vi "SSIToolMain.vi"() -> ()   [LabVIEW 2019]
uses:
  testSeq/TestSeqClass.lvclass
  Exe_Queues/TypeDef/mainExeStates.ctl
  Exe_Queues/TypeDef/mainEventInfo.ctl
  GUIHandler/GUI_Handler_Seq.lvclass
  GUIHandler_Main/GUI_Handler_Main.lvclass
  GUIHandler/GuiSectionEnum.ctl
  Typedef/TestTypeSelect.ctl
  ProgramSettings/ProgramSettings.lvclass
panel:
  in  "Calibration_ListBox":i32(listbox)=-1
  in  "Operatør beskeder":T1={"Operator_Aceept"=FALSE, "Operator_decline "=FALSE, "User message "="Er Lysdioden slukket"}
  in  "Forsyningsspænding":u16(ring)=1 items=["", "5V", "9 - 30 V"]
  out "Calibration Status":bool=TRUE
  out "Multiturn værdi":dbl
  out "Singleturn værdi":dbl
  out "Test Status":bool=TRUE
  in  "Test_Listbox":i32(listbox)=-1
  in  "Kode":u16(ring)=2 items=["", "Binær", "Gray"]
  in  "Opløsning":u16(ring)=2 items=["", "0013", "1213", "1613", "2013", "2413"]
  in  "Konfigurations Filnavn":string="Test.cfg"
  out "Dial":dbl(knob)=0.604351805313778 scale=0.0..360.0
  in  "StartCalibration":bool
  in  "StartAfprøvning":bool
  in  "Start Alt":bool
  in  "Stop":bool
  # "Variant setup"
  # "Konfiguration"
  # "Afprøvning"
  # "Aktuelle værdier"
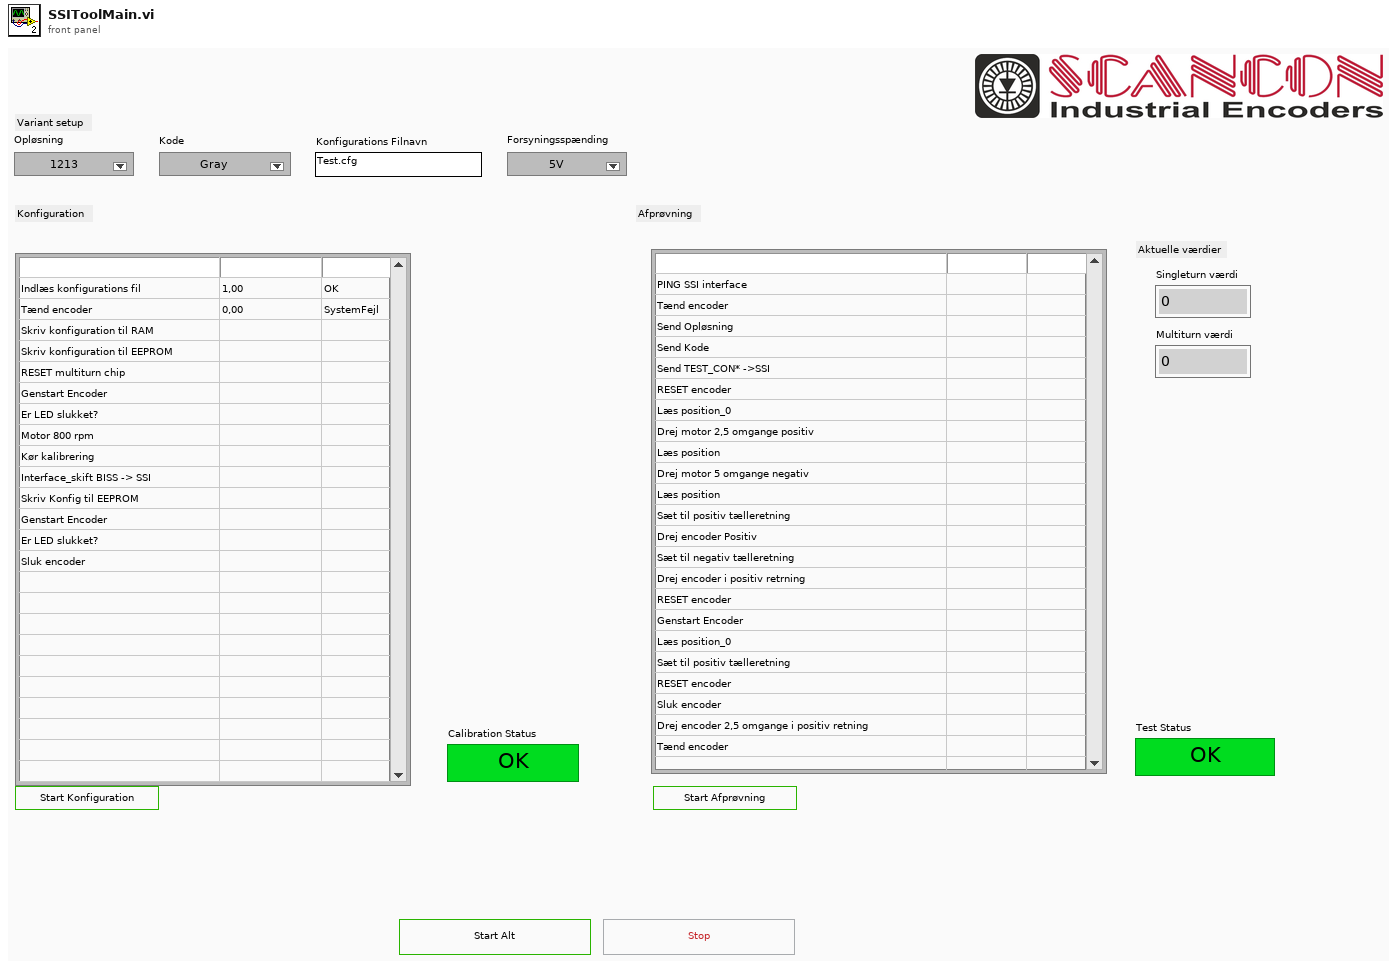
[diagram p1: front panel]
types:
  T1 = cluster{"Operator_Aceept":bool, "Operator_decline ":bool, "User message ":string}
  T2 = cluster{"Start Alt":refnum<vi>, "Stop":refnum<vi>, "Operatør beskeder":refnum<vi>}
  T3 = typedef "GuiSectionEnum.ctl" = enum16{"TestingSection", "CalibrationSection"}
  T4 = cluster{"Konfigurations Filnavn":refnum<vi>, "Forsyningsspænding":refnum<vi>, "Kode":refnum<vi>, "Opløsning":refnum<vi>}
  T5 = typedef "mainEventInfo.ctl" = cluster{"MainExeStates":T6, "Data":variant}
  T6 = typedef "mainExeStates.ctl" = enum16{"Idle", "Load_Seq_File", "Save_Seq_File", "Init", "StartKalib", "StartAfprøvning", "StartAlt", "Stop", "Exit", "SettingsDialog", "Update_Config_FileName", "Seq_Calibrate_setup"}
  T7 = cluster{"Multiturn værdi":refnum<vi>, "Singleturn værdi":refnum<vi>, "Test Status":refnum<vi>, "Test_Listbox":refnum<vi>, "Dial":refnum<vi>, "StartAfprøvning":refnum<vi>}
  T8 = typedef "TestTypeSelect.ctl" = enum16{"Calibration", "Testing"}
  T9 = cluster{"MHM_Handle out":u32, "axis out":cluster{"keyHandle":u32, "nodeId":u16}}
  T10 = enum32{"invalid app kind", "Development System", "Run Time System", "Student Edition", "Embedded LabVIEW", "Evaluation", "Custom"}
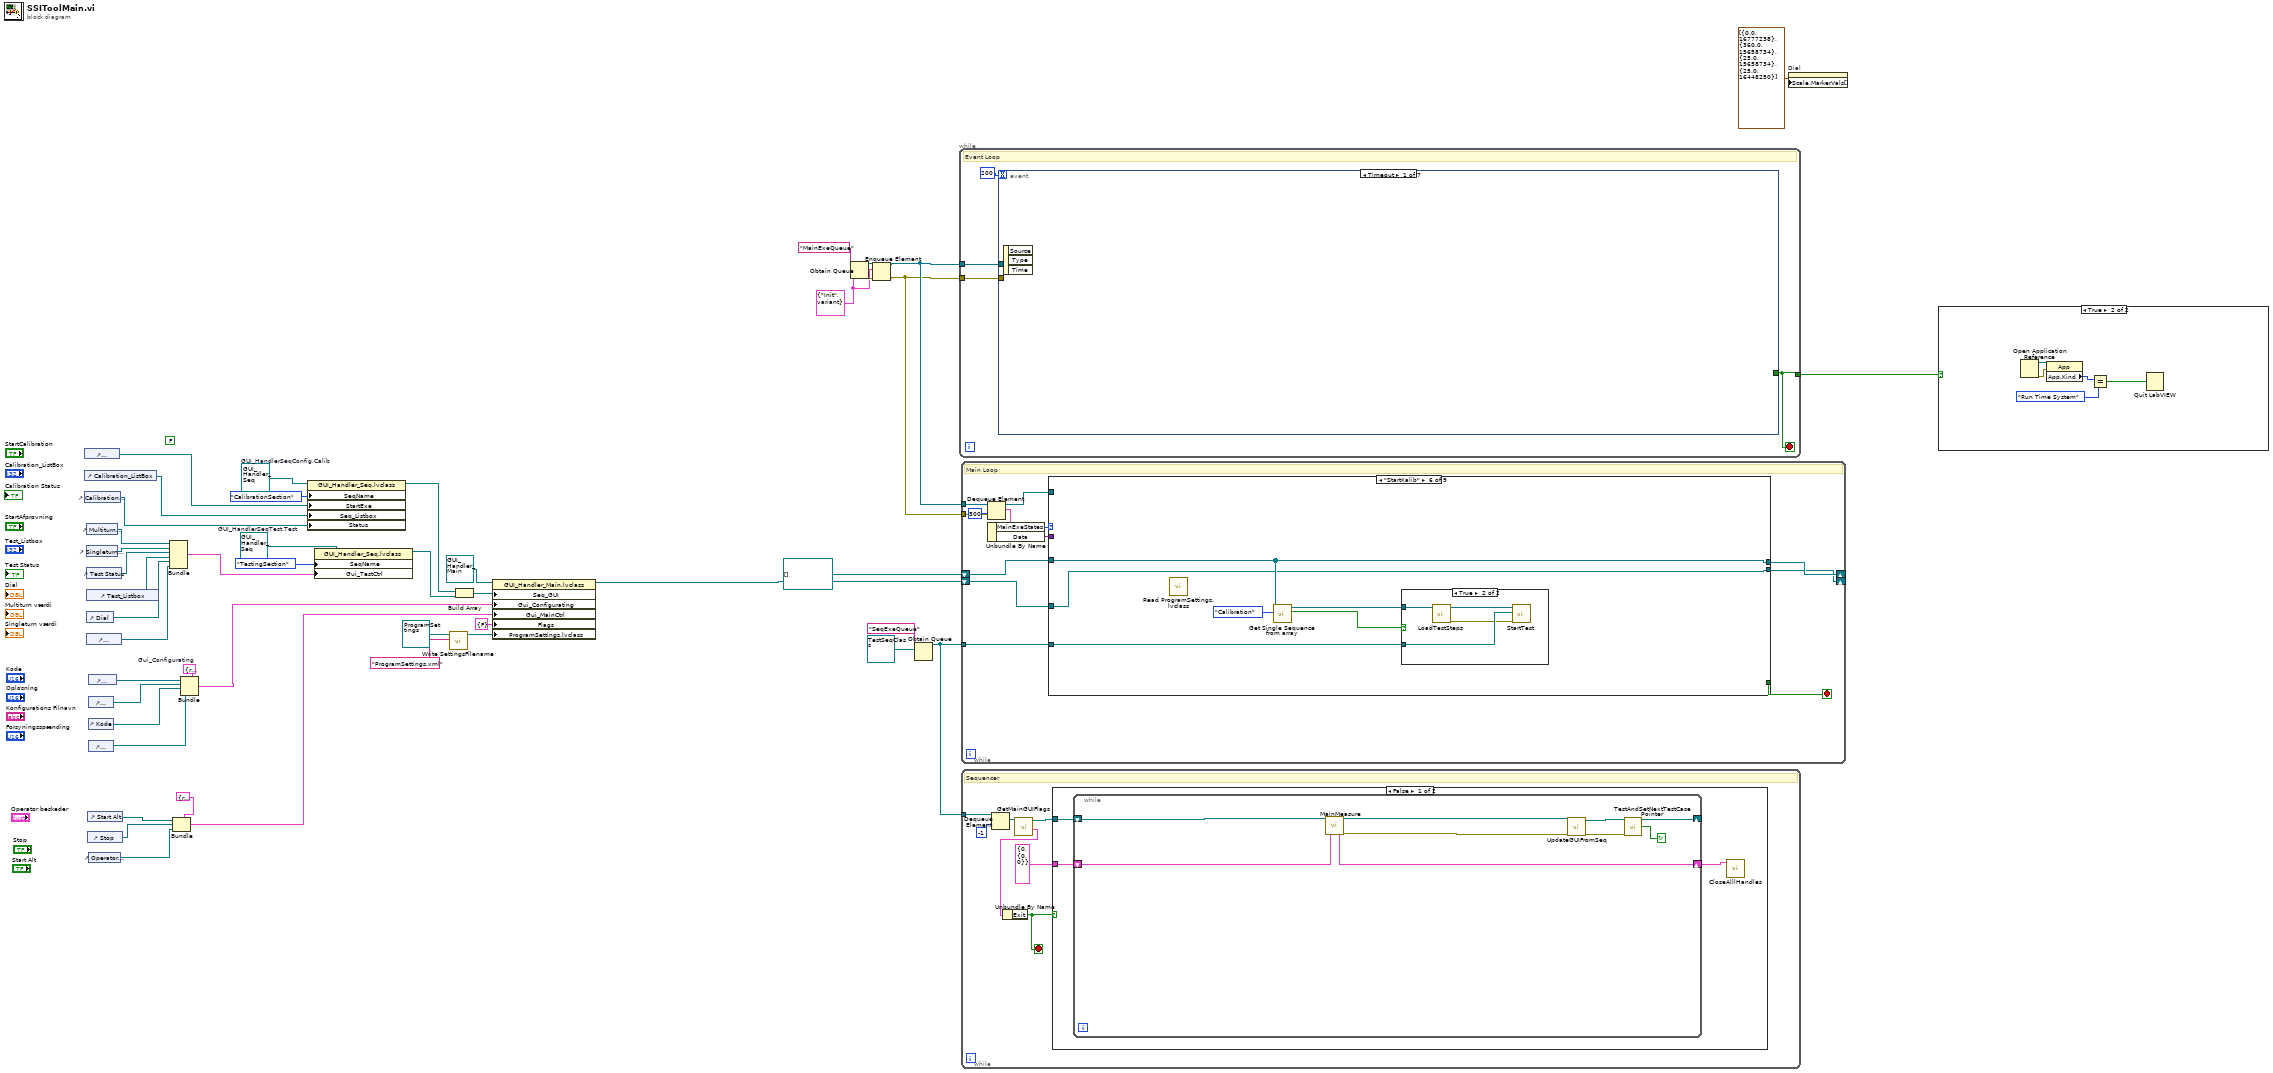
[diagram p0: block diagram]
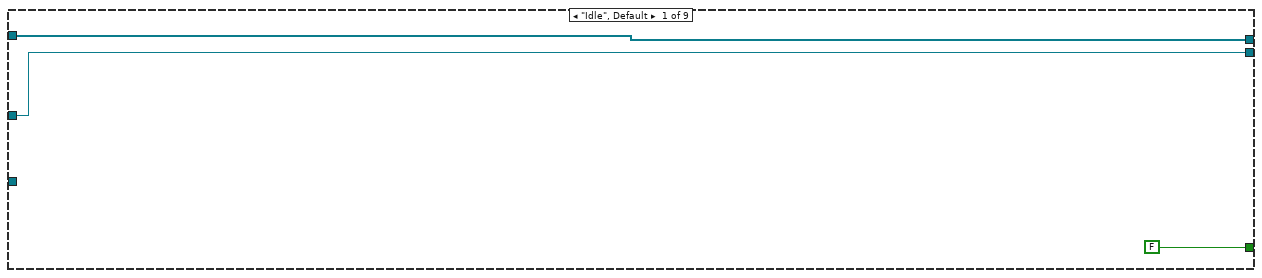
[diagram p4: hidden frame]
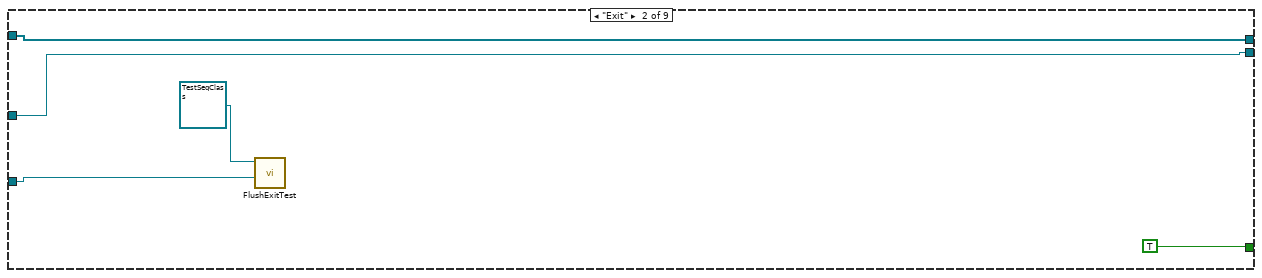
[diagram p5: hidden frame]
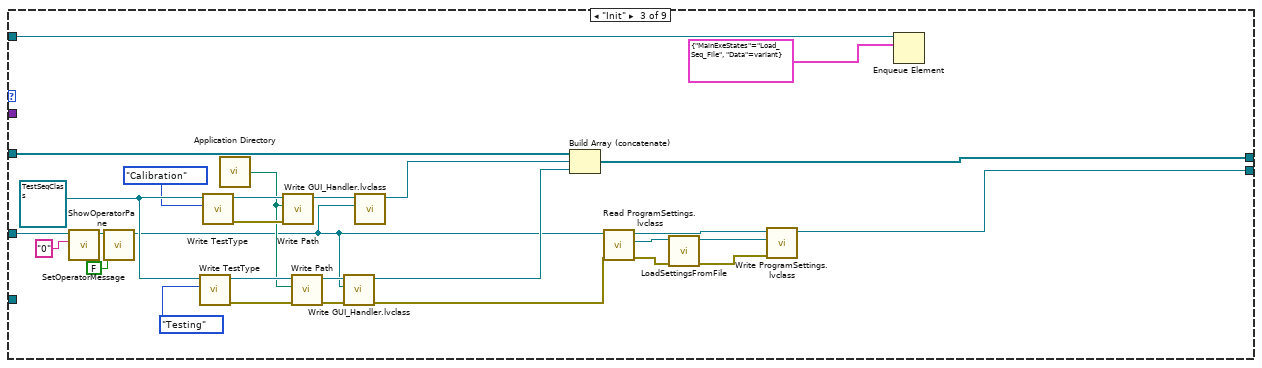
[diagram p6: hidden frame]
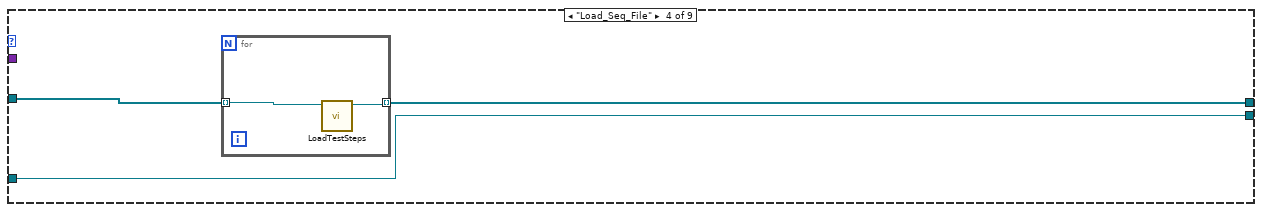
[diagram p7: hidden frame]
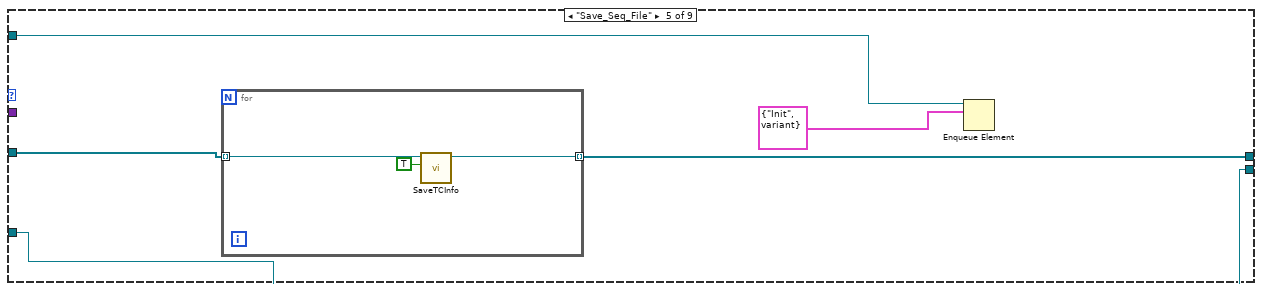
[diagram p8: hidden frame]
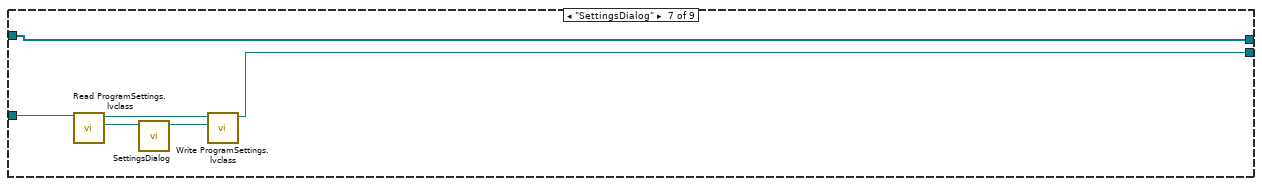
[diagram p10: hidden frame]
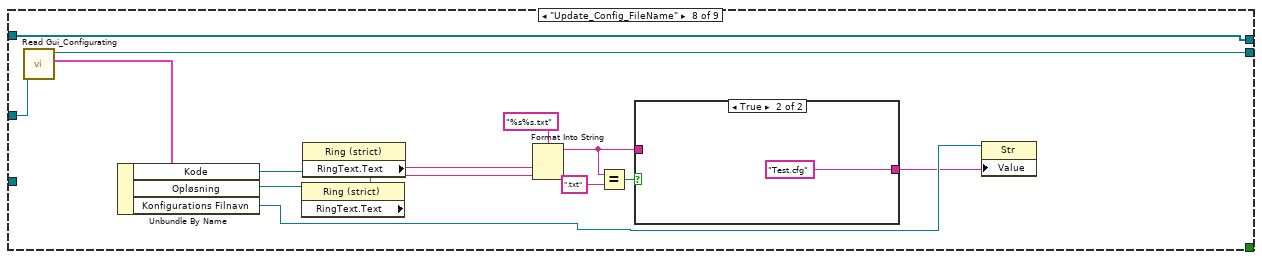
[diagram p11: hidden frame]
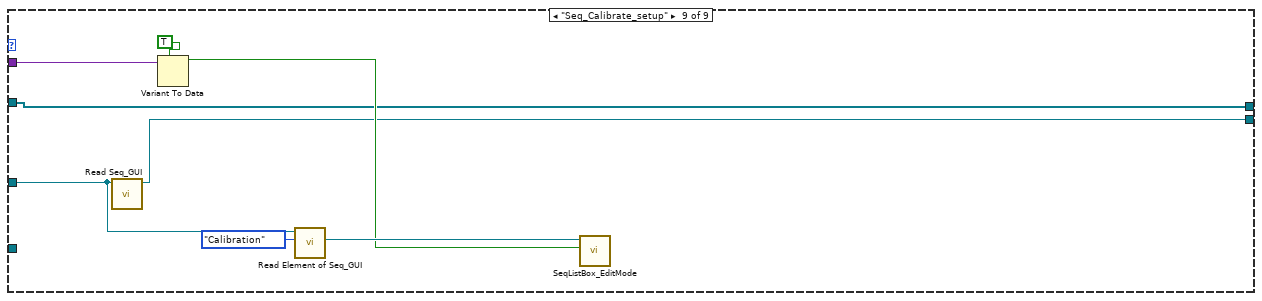
[diagram p13: hidden frame]
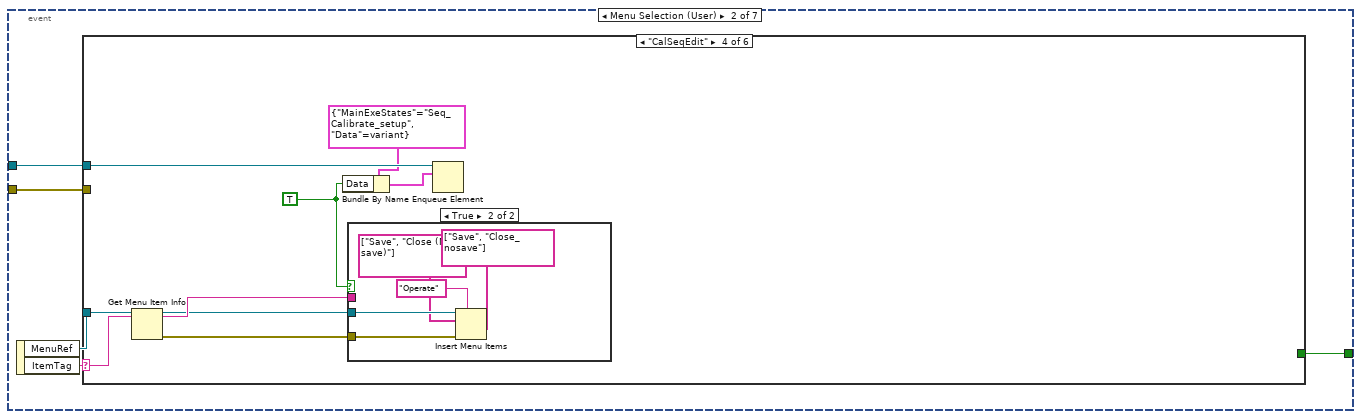
[diagram p14: hidden frame]
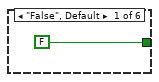
[diagram p15: hidden frame]
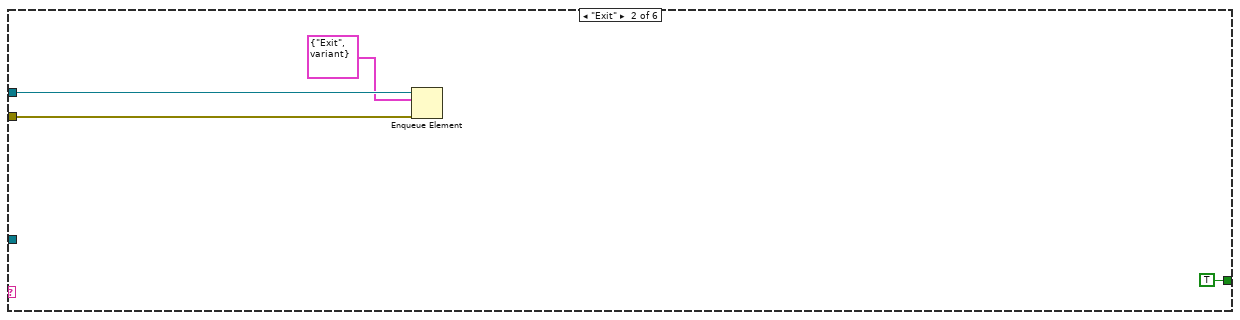
[diagram p16: hidden frame]
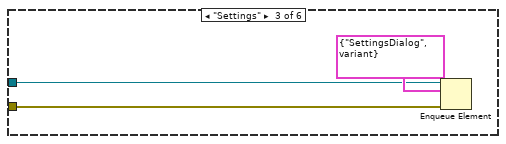
[diagram p17: hidden frame]
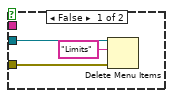
[diagram p18: hidden frame]
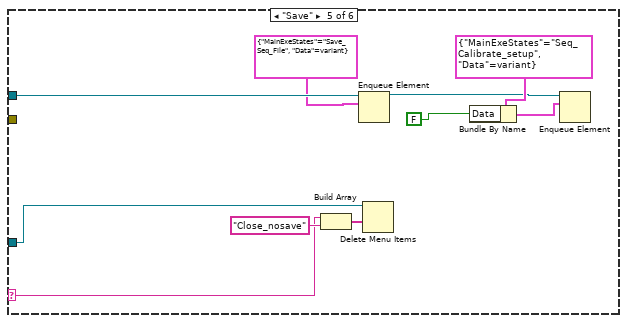
[diagram p19: hidden frame]
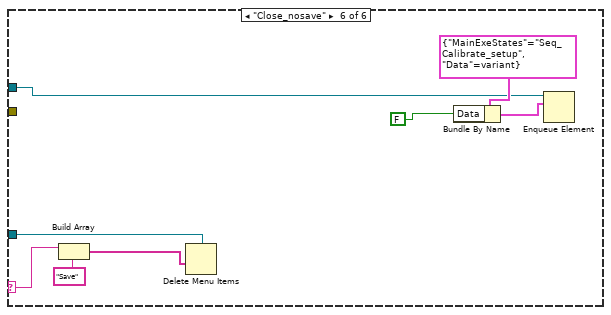
[diagram p20: hidden frame]
diagram:
  (unwired) FALSE ("Blinking")
  w26 = T4 {"Konfigurations Filnavn"=refnum, "Forsyningsspænding"=refnum, "Kode"=refnum, "Opløsning"=refnum}  # Gui_Configurating
  w20 = refnum<class "GUI_Handler_Seq.lvclass"> refnum  # GUI_HandlerSeqTest.Test
  w39 = T5 {"MainExeStates"=enum."Init", "Data"=variant}
  w25 = refnum<class "GUI_Handler_Seq.lvclass"> refnum  # GUI_HandlerSeqConfig.Calib
  n1 = control-ref of="StartCalibration"() -> (w23:refnum<vi>)
  n2 = control-ref of="Calibration_ListBox"() -> (w22:refnum<vi>)
  n3 = control-ref of="Calibration Status"() -> (w10:refnum<vi>)
  n4 = control-ref of="Multiturn værdi"() -> (w32:refnum<vi>)
  n5 = control-ref of="Singleturn værdi"() -> (w31:refnum<vi>)
  n6 = control-ref of="Test Status"() -> (w30:refnum<vi>)
  n7 = control-ref of="Test_Listbox"() -> (w29:refnum<vi>)
  n8 = control-ref of="Dial"() -> (w28:refnum<vi>)
  n9 = control-ref of="StartAfprøvning"() -> (w27:refnum<vi>)
  n10 = control-ref of="Stop"() -> (w3:refnum<vi>)
  n11 = control-ref of="Start Alt"() -> (w4:refnum<vi>)
  n12 = control-ref of="Konfigurations Filnavn"() -> (w36:refnum<vi>)
  n13 = control-ref of="Forsyningsspænding"() -> (w35:refnum<vi>)
  n14 = control-ref of="Kode"() -> (w34:refnum<vi>)
  n15 = control-ref of="Opløsning"() -> (w33:refnum<vi>)
  n16 = control-ref of="Operatør beskeder"() -> (w2:refnum<vi>)
  n17 = Bundle("Multiturn værdi"=w32, "Singleturn værdi"=w31, "Test Status"=w30, "Test_Listbox"=w29, "Dial"=w28, "StartAfprøvning"=w27) -> (w19:T7)  [unwired: 1 in]
  n18 = Bundle(cluster=T2 {"Start Alt"=refnum, "Stop"=refnum, "Operatør beskeder"=refnum} ("output cluster"), "Start Alt"=w4, "Stop"=w3, "Operatør beskeder"=w2) -> (w5:T2)
  n19 = Bundle(cluster=w26, "Konfigurations Filnavn"=w36, "Forsyningsspænding"=w35, "Kode"=w34, "Opløsning"=w33) -> (w16:T4)
  n20 = property class="GUI_Handler_Seq.lvclass"(reference=w25, "SeqName"=GuiSectionEnum."CalibrationSection", "StartExe"=w23, "Seq_Listbox"=w22, "Status"=w10) -> (reference out=w43:refnum<class "GUI_Handler_Seq.lvclass">)  [unwired: 1 in, 1 out]
  n21 = property class="GUI_Handler_Seq.lvclass"(reference=w20, "SeqName"=GuiSectionEnum."TestingSection", "Gui_TestCtrl"=w19) -> (reference out=w42:refnum<class "GUI_Handler_Seq.lvclass">)  [unwired: 1 in, 1 out]
  n22 = call "Write SettingsFilename.vi"("SettingsFilename"="ProgramSettings.xml", "ProgramSettings in"=refnum<class "ProgramSettings.lvclass"> refnum ("ProgramSettings.lvclass")) -> ("ProgramSettings out"=w7:refnum<class "ProgramSettings.lvclass">)  [unwired: 8 in, 1 out]
  n23 = Build Array(w43, w42) -> (w17:refnum<class "GUI_Handler_Seq.lvclass">[])
  n24 = property class="GUI_Handler_Main.lvclass"(reference=refnum<class "GUI_Handler_Main.lvclass"> refnum ("GUI_Handler_Main.lvclass"), "Seq_GUI"=w17, "Gui_Configurating"=w16, "Gui_MainCtrl"=w5, "Flags"=cluster{"Exit":bool} {"Exit"=FALSE}, "ProgramSettings.lvclass"=w7) -> (reference out=w15:refnum<class "GUI_Handler_Main.lvclass">)  [unwired: 1 in, 1 out]
  n25 = Obtain Queue(name (unnamed)="MainExeQueue", element data type=w39) -> (queue out=w41:refnum<queue>, error out=w40:errorcluster)  [unwired: 3 in, 1 out]
  n26 = Enqueue Element(queue=w41, element=w39, error in (no error)=w40) -> (queue out=w38:refnum<queue>, error out=w37:errorcluster)  [unwired: 1 in, 1 out]
  n27 = Obtain Queue(name (unnamed)="SeqExeQueue", element data type=refnum<class "TestSeqClass.lvclass"> refnum ("TestSeqClass.lvclass")) -> (queue out=w11:refnum<queue>)  [unwired: 3 in, 2 out]
  n28 = while {
    tunnel: [w49] -> w45
    tunnel: w38 -> [w48]
    tunnel: w37 -> [w47]
    stop <- w49 stop-if-true
    # "Event Loop"
    n29 = event shown="[0] Timeout" {
      selector: _ -> [_ _ _ _ _ _ _]
      dyn-events: _ -> [_ _ _ _ _ _ _]
      timeout: 200 -> [_ _ _ _ _ _ _]
      tunnel: [_ w54 _ _ _ _ _] -> w49
      tunnel: w48 -> [_ w53 w99 w101 w104 w110 _]
      tunnel: w47 -> [_ w52 w98 _ w103 w109 _]
      event Timeout {
        n30 = event-data() -> ()  [unwired: 1 in, 3 out]
      }
      event Menu Selection (User) {
        n31 = event-data() -> ("MenuRef"=w51:refnum<k9>, "ItemTag"=w55:string)  [unwired: 1 in]
        n32 = case shown="\"CalSeqEdit\"" w55 {
          selector: w55 -> [_ _ _ w67 w85 w92]
          tunnel: [FALSE TRUE _ _ _ _] -> w54
          tunnel: w53 -> [_ w59 w62 w71 w89 w96]
          tunnel: w52 -> [_ w58 w61 _ _ _]
          tunnel: w51 -> [_ _ _ w70 w84 w93]
          frame "False", Default {
          }
          frame "Exit" {
            n33 = Enqueue Element(queue=w59, element=T5 {"MainExeStates"=enum."Exit", "Data"=variant}, error in (no error)=w58) -> ()  [unwired: 1 in, 3 out]
          }
          frame "Settings" {
            n34 = Enqueue Element(queue=w62, element=T5 {"MainExeStates"=enum."SettingsDialog", "Data"=variant}, error in (no error)=w61) -> ()  [unwired: 1 in, 3 out]
          }
          frame "CalSeqEdit" {
            w64 = TRUE
            n35 = Get Menu Item Info(7:w67, 11:w70) -> (0:w65:errorcluster, 3:w66:refnum<k9>)  [unwired: 1 in, 5 out]
            n36 = Bundle By Name(cluster=T5 {"MainExeStates"=enum."Seq_Calibrate_setup", "Data"=variant} ("element"), "Data"=w64) -> (w68:T5)
            n37 = case shown="True" w64 {
              tunnel: w65 -> [w74 w79]
              tunnel: w66 -> [w73 w78]
              tunnel: w67 -> [_ _]
              frame False {
                n38 = Delete Menu Items(6:w74, 8:"Limits" ("menu tag"), 9:w73) -> ()  [unwired: 1 in, 2 out]
              }
              frame True {
                n39 = Insert Menu Items(5:"Operate" ("menu tag"), 6:w79, 7:string[] ["Save", "Close_nosave"] ("item tags"), 8:string[] ["Save", "Close (No save)"] ("item names"), 9:w78) -> ()  [unwired: 1 in, 3 out]
              }
            }
            n40 = Enqueue Element(queue=w71, element=w68) -> ()  [unwired: 2 in, 3 out]
          }
          frame "Save" {
            n41 = Build Array(w85, "Close_nosave" ("element")) -> (w87:string[])
            n42 = Enqueue Element(queue=w89, element=T5 {"MainExeStates"=enum."Save_Seq_File", "Data"=variant}) -> (queue out=w80:refnum<queue>)  [unwired: 2 in, 2 out]
            n43 = Delete Menu Items(7:w87, 9:w84) -> ()  [unwired: 2 in, 2 out]
            n44 = Bundle By Name(cluster=T5 {"MainExeStates"=enum."Seq_Calibrate_setup", "Data"=variant} ("element"), "Data"=FALSE) -> (w81:T5)
            n45 = Enqueue Element(queue=w80, element=w81) -> ()  [unwired: 2 in, 3 out]
          }
          frame "Close_nosave" {
            n46 = Build Array(w92, "Save" ("element")) -> (w91:string[])
            n47 = Delete Menu Items(7:w91, 9:w93) -> ()  [unwired: 2 in, 2 out]
            n48 = Bundle By Name(cluster=T5 {"MainExeStates"=enum."Seq_Calibrate_setup", "Data"=variant} ("element"), "Data"=FALSE) -> (w94:T5)
            n49 = Enqueue Element(queue=w96, element=w94) -> ()  [unwired: 2 in, 3 out]
          }
        }
      }
      event "Opløsning", "Kode": Value Change {
        n50 = event-data() -> ()  [unwired: 1 in, 5 out]
        n51 = Enqueue Element(queue=w99, element=T5 {"MainExeStates"=enum."Update_Config_FileName", "Data"=variant}, error in (no error)=w98) -> ()  [unwired: 1 in, 3 out]
      }
      event "StartAfprøvning": Value Change {
        n52 = event-data() -> ()  [unwired: 1 in, 5 out]
        n53 = Enqueue Element(queue=w101, element=T5 {"MainExeStates"=enum."StartAfprøvning", "Data"=variant}) -> ()  [unwired: 2 in, 3 out]
      }
      event "StartCalibration": Value Change {
        n54 = event-data() -> ()  [unwired: 1 in, 5 out]
        n55 = Enqueue Element(queue=w104, element=T5 {"MainExeStates"=enum."StartKalib", "Data"=variant}, error in (no error)=w103) -> ()  [unwired: 1 in, 3 out]
      }
      event "Start Alt": Value Change {
        n56 = event-data() -> ()  [unwired: 1 in, 5 out]
        n57 = Enqueue Element(queue=w110, element=T5 {"MainExeStates"=enum."StartKalib", "Data"=variant}, error in (no error)=w109) -> (queue out=w107:refnum<queue>, error out=w106:errorcluster)  [unwired: 1 in, 1 out]
        n58 = Enqueue Element(queue=w107, element=T5 {"MainExeStates"=enum."StartAfprøvning", "Data"=variant}, error in (no error)=w106) -> ()  [unwired: 1 in, 3 out]
      }
      event "Operatør beskeder.Operator_Aceept": Value Change {
        n59 = event-data() -> ()  [unwired: 1 in, 5 out]
      }
    }
  }
  n60 = while {
    tunnel: w38 -> [w124]
    tunnel: w37 -> [w123]
    shift-right: [w119] -> _
    shift-left: refnum<class "TestSeqClass.lvclass">[] [] -> [w120]
    tunnel: w11 -> [w114]
    shift-right: [w113] -> _
    shift-left: w15 -> [w116]
    stop <- w115 stop-if-true
    # "Main Loop"
    n61 = Dequeue Element(queue=w124, timeout in ms (-1)=500, error in (no error)=w123) -> (queue out=w118:refnum<queue>, element=w122:T5)  [unwired: 2 out]
    n62 = Unbundle By Name(w122) -> ("MainExeStates"=w121:T6, "Data"=w112:variant)
    n63 = case shown="\"StartKalib\"" w121 {
      tunnel: w120 -> [w127 w129 w152 w164 w167 w179 w185 w191 w208]
      tunnel: [w127 w129 w158 w163 w168 w179 w185 w191 w208] -> w119
      tunnel: w118 -> [_ _ w153 _ w169 _ _ _ _]
      tunnel: w116 -> [w125 w128 w137 w162 w171 w175 w190 w204 w214]
      tunnel: [FALSE TRUE _ _ _ _ _ _ _] -> w115
      tunnel: w114 -> [_ w131 _ _ _ w180 _ _ _]
      tunnel: [w125 w128 w141 w162 w171 w175 w186 w198 w207] -> w113
      tunnel: w112 -> [_ _ _ _ _ _ _ _ w211]
      frame "Idle", Default {
      }
      frame "Exit" {
        n64 = call-dynamic "FlushExitTest.vi"("SeqExeQuueIn"=w131, "TestSeqClass in"=refnum<class "TestSeqClass.lvclass"> refnum) -> ()  [unwired: 8 in, 2 out]
      }
      frame "Init" {
        w157 = refnum<class "TestSeqClass.lvclass"> refnum ("TestSeqClass.lvclass")
        n65 = call-dynamic "SetOperatorMessage.vi"("Value"="0", "GUI_Handler_Main in"=w137) -> ("GUI_Handler_Main out"=w134:refnum<class "GUI_Handler_Main.lvclass">)  [unwired: 8 in, 1 out]
        n66 = call-dynamic "ShowOperatorPane.vi"("Visible"=FALSE, "GUI_Handler_Main in"=w134) -> ("GUI_Handler_Main out"=w133:refnum<class "GUI_Handler_Main.lvclass">)  [unwired: 8 in, 1 out]
        n67 = call-dynamic "Write TestType.vi"("TestType"=TestTypeSelect."Testing", "TestSeqClass in"=w157) -> ("error out"=w155:errorcluster, "TestSeqClass out"=w159:refnum<class "TestSeqClass.lvclass">)  [unwired: 8 in]
        n68 = call-dynamic "Write TestType.vi"("TestType"=TestTypeSelect."Calibration", "TestSeqClass in"=w157) -> ("error out"=w160:errorcluster, "TestSeqClass out"=w161:refnum<class "TestSeqClass.lvclass">)  [unwired: 8 in]
        n69 = call <vilib>:"Application Directory.vi"() -> ("Application Directory"=w156:path)
        n70 = call-dynamic "Write Path.vi"("error in (no error)"=w160, "Path"=w156, "TestSeqClass in"=w161) -> ("TestSeqClass out"=w149:refnum<class "TestSeqClass.lvclass">)  [unwired: 7 in, 1 out]
        n71 = call-dynamic "Write Path.vi"("error in (no error)"=w155, "Path"=w156, "TestSeqClass in"=w159) -> ("error out"=w145:errorcluster, "TestSeqClass out"=w148:refnum<class "TestSeqClass.lvclass">)  [unwired: 7 in]
        n72 = call-dynamic "Write GUI_Handler.lvclass.vi"("error in (no error)"=w145, "GUI_Handler.lvclass"=w133, "TestSeqClass in"=w148) -> ("error out"=w139:errorcluster, "TestSeqClass out"=w147:refnum<class "TestSeqClass.lvclass">)  [unwired: 7 in]
        n73 = call-dynamic "Write GUI_Handler.lvclass.vi"("GUI_Handler.lvclass"=w133, "TestSeqClass in"=w149) -> ("TestSeqClass out"=w146:refnum<class "TestSeqClass.lvclass">)  [unwired: 8 in, 1 out]
        n74 = Build Array (concatenate)(w152, w146, w147) -> (w158:refnum<class "TestSeqClass.lvclass">[])
        n75 = call "Read ProgramSettings.lvclass.vi"("error in (no error)"=w139, "GUI_Handler_Main in"=w133) -> ("error out"=w140:errorcluster, "ProgramSettings.lvclass"=w143:refnum<class "ProgramSettings.lvclass">, "GUI_Handler_Main out"=w144:refnum<class "GUI_Handler_Main.lvclass">)  [unwired: 7 in]
        n76 = call "LoadSettingsFromFile.vi"("error in (no error)"=w140, "ProgramSettings in"=w143) -> ("error out"=w138:errorcluster, "ProgramSettings out"=w142:refnum<class "ProgramSettings.lvclass">)  [unwired: 8 in]
        n77 = call "Write ProgramSettings.lvclass.vi"("error in (no error)"=w138, "ProgramSettings.lvclass"=w142, "GUI_Handler_Main in"=w144) -> ("GUI_Handler_Main out"=w141:refnum<class "GUI_Handler_Main.lvclass">)  [unwired: 7 in, 1 out]
        n78 = Enqueue Element(queue=w153, element=T5 {"MainExeStates"=enum."Load_Seq_File", "Data"=variant}) -> ()  [unwired: 2 in, 3 out]
      }
      frame "Load_Seq_File" {
        n79 = for {
          tunnel: w164 -> [w166] mode=indexing
          tunnel: [w165] -> w163 mode=indexing
          n80 = call-dynamic "LoadTestSteps.vi"("TestSeqClass in"=w166) -> ("TestSeqClass out"=w165:refnum<class "TestSeqClass.lvclass">)  [unwired: 9 in, 1 out]
        }
      }
      frame "Save_Seq_File" {
        n81 = for {
          tunnel: w167 -> [w174] mode=indexing
          tunnel: [w172] -> w168 mode=indexing
          n82 = call "SaveTCInfo.vi"("Save"=TRUE, "TestSeqClass.lvclass"=w174) -> ("TestSeqClass out"=w172:refnum<class "TestSeqClass.lvclass">)  [unwired: 8 in, 1 out]
        }
        n83 = Enqueue Element(queue=w169, element=T5 {"MainExeStates"=enum."Init", "Data"=variant}) -> ()  [unwired: 2 in, 3 out]
      }
      frame "StartKalib" {
        n84 = call "Read ProgramSettings.lvclass.vi"() -> ()  [unwired: 9 in, 3 out]
        n85 = call "Get Single Sequence from array.vi"("TestType"=TestTypeSelect."Calibration", "Sequences"=w179) -> ("Found"=w178:bool, "TestSeqClass.lvclass"=w176:refnum<class "TestSeqClass.lvclass">)  [unwired: 7 in, 1 out]
        n86 = case shown="True" w178 {
          tunnel: w176 -> [_ w183]
          tunnel: w180 -> [_ w184]
          frame False {
          }
          frame True {
            n87 = call-dynamic "LoadTestSteps.vi"("TestSeqClass in"=w183) -> ("error out"=w181:errorcluster, "TestSeqClass out"=w182:refnum<class "TestSeqClass.lvclass">)  [unwired: 9 in]
            n88 = call-dynamic "StartTest.vi"("error in (no error)"=w181, "SeqExeQuueIn"=w184, "TestSeqClass in"=w182) -> ()  [unwired: 7 in, 2 out]
          }
        }
      }
      frame "SettingsDialog" {
        n89 = call "Read ProgramSettings.lvclass.vi"("GUI_Handler_Main in"=w190) -> ("ProgramSettings.lvclass"=w189:refnum<class "ProgramSettings.lvclass">, "GUI_Handler_Main out"=w187:refnum<class "GUI_Handler_Main.lvclass">)  [unwired: 8 in, 1 out]
        n90 = call "SettingsDialog.vi"("ProgramSettings in"=w189) -> ("ProgramSettings out"=w188:refnum<class "ProgramSettings.lvclass">)  [unwired: 9 in, 1 out]
        n91 = call "Write ProgramSettings.lvclass.vi"("ProgramSettings.lvclass"=w188, "GUI_Handler_Main in"=w187) -> ("GUI_Handler_Main out"=w186:refnum<class "GUI_Handler_Main.lvclass">)  [unwired: 8 in, 1 out]
      }
      frame "Update_Config_FileName" {
        n92 = call-dynamic "Read Gui_Configurating.vi"("GUI_Handler_Main in"=w204) -> ("Gui_Configurating"=w199:T4, "GUI_Handler_Main out"=w198:refnum<class "GUI_Handler_Main.lvclass">)  [unwired: 8 in, 1 out]
        n93 = Unbundle By Name(w199) -> ("Kode"=w203:refnum<vi>, "Opløsning"=w202:refnum<vi>, "Konfigurations Filnavn"=w193:refnum<vi>)
        n94 = property class="Ring (strict)"(reference=w202) -> ("RingText.Text"=w201:string)  [unwired: 1 in, 2 out]
        n95 = property class="Ring (strict)"(reference=w203) -> ("RingText.Text"=w197:string)  [unwired: 1 in, 2 out]
        n96 = Format Into String(format string="%s%s.txt", w197, w201) -> (resulting string=w196:string)  [unwired: 2 in, 1 out]
        n97 = Equal?(x=w196, y=".txt") -> (x = y?=w194:bool)
        n98 = case shown="True" w194 {
          tunnel: w196 -> [w205 _]
          tunnel: [w205 "Test.cfg" ("Value")] -> w192
          frame False {
          }
          frame True {
          }
        }
        n99 = property class="Str"(reference=w193, "Value"=w192) -> ()  [unwired: 1 in, 2 out]
      }
      frame "Seq_Calibrate_setup" {
        n100 = call-dynamic "Read Seq_GUI.vi"("GUI_Handler_Main in"=w214) -> ("GUI_Handler_Main out"=w207:refnum<class "GUI_Handler_Main.lvclass">)  [unwired: 8 in, 2 out]
        n101 = Variant To Data(type=TRUE, Variant=w211) -> (data=w209:bool)  [unwired: 1 in, 1 out]
        n102 = call-dynamic "Read Element of Seq_GUI.vi"("Variant"=TestTypeSelect."Calibration", "GUI_Handler_Main in"=w214) -> ("GUI_Handler_Seq.lvclass"=w212:refnum<class "GUI_Handler_Seq.lvclass">)  [unwired: 7 in, 2 out]
        n103 = call-dynamic "SeqListBox_EditMode.vi"("Debug"=w209, "GUI_Handler_Seq in"=w212) -> ()  [unwired: 8 in, 2 out]
      }
    }
  }
  n104 = while {
    tunnel: w11 -> [w220]
    stop <- w219 stop-if-true
    # "Sequencer"
    n105 = Dequeue Element(queue=w220, timeout in ms (-1)=-1) -> (element=w218:refnum<class "TestSeqClass.lvclass">)  [unwired: 1 in, 3 out]
    n106 = call-dynamic "GetMainGUIFlags.vi"("TestSeqClass in"=w218) -> ("Flags"=w216:cluster{"Exit":bool}, "TestSeqClass out"=w217:refnum<class "TestSeqClass.lvclass">)  [unwired: 8 in, 1 out]
    n107 = Unbundle By Name(w216) -> ("Exit"=w219:bool)
    n108 = case shown="False" w219 {
      tunnel: w217 -> [w224 _]
      tunnel: T9 {"MHM_Handle out"=0, "axis out"={"keyHandle"=0, "nodeId"=0}} ("Handles_Out") -> [w223 _]
      frame False {
        n109 = while {
          shift-right: [w231] -> _
          shift-left: w224 -> [w229]
          shift-right: [w225] -> w222
          shift-left: w223 -> [w226]
          stop <- w233 continue-if-true
          n110 = call "MainMeasure.vi"("TestSeqClass.lvclass"=w229, "Handles_In"=w226) -> ("Handles_Out"=w225:T9, "TestSeqClass out"=w228:refnum<class "TestSeqClass.lvclass">, "error out"=w227:errorcluster)  [unwired: 14 in, 1 out]
          n111 = call "UpdateGUIFromSeq.vi"("TestSeqClass in"=w228, "error in (no error)"=w227) -> ("TestSeqClass out"=w232:refnum<class "TestSeqClass.lvclass">, "error out"=w230:errorcluster)  [unwired: 12 in]
          n112 = call "TestAndSetNextTestCasePointer.vi"("TestSeqClass in"=w232, "error in (no error)"=w230) -> ("TestSeqClass out"=w231:refnum<class "TestSeqClass.lvclass">, "Continue"=w233:bool)  [unwired: 10 in, 2 out]
        }
        n113 = call "CloseAlllHandles.vi"("Handles_In"=w222) -> ()  [unwired: 9 in, 2 out]
      }
      frame True {
      }
    }
  }
  n114 = property on="Dial" class="Knob (strict)"("Scale.MarkerVals[]"=cluster{dbl, u32}[] [{0.0, 16777238}, {360.0, 15658734}, {25.0, 15658734}, {25.0, 16448250}] ("Scale.Marker Values[]")) -> ()  [unwired: 2 in, 2 out]
  n115 = case shown="True" w45 {
    frame False {
    }
    frame True {
      n116 = Open Application Reference() -> (0:w238:errorcluster, 3:w237:refnum<vi>)  [unwired: 4 in]
      n117 = property class="App"(reference=w237, error in=w238) -> ("App.Kind"=w236:T10)  [unwired: 2 out]
      n118 = Equal?(x=w236, y=T10."Run Time System") -> (x = y?=w234:bool)
      n119 = Quit LabVIEW(quit? (T)=w234) -> ()
    }
  }
